vi "Emballae_BDD_Tableau pièces emballées ds GPAO.vi"(8 "error in (no error)":errorcluster caption="entrée d'erreur (pas d'erreur)", 9 "Code bar fixe avec indice":string="1121057400", 11 "connection information":path=path "\\\\Plz-inf-nas\\medic/PARAMETRES_TESTS/PROD_Data-Admin/Connection.udl") -> (0 "error out":errorcluster, 2 "Erreur de\n comunication":bool, 3 "Tableau historique":string[][](array[string])=[["112105740008090004", "01.01.2001 01:01:00", "55", "01234/08-01.01.01", "1", "0"], ["112105740008090006", "01.01.2001 01:01:00", "55", "56789/08-01.01.01", "3", "0"], ["112105740008090007", "01.01.2001 01:01:00", "55", "56789/08-01.01.01", "4", "0"], ["112105740008090007", "01.01.2001 01:01:00", "55", "00123/08-01.01.01", "2", "1"]])   [LabVIEW 2020]
doc: "Renvoie l'historique des articlesidentiques à celui scanné et déjà emballés d'après la GPAO.\nLe tableau historique contient les données suivantes :\n colonne 0 : n° des pièces (code bar 18 chiffres)\n colonne 1 : date\n colonne 2 : visa emballage (n°)\n colonne 3 : n° commande (complet)\n colonne 4 : n° carton\n colonne 5 : n° retour (0, pas un retour)"
uses:
  Modules/FS/60_FS_Controles/60_FS_SetGet.ctl
  <vilib>/addons/database/Connection.llb/DB Tools Open Connec (Path).vi
  <vilib>/addons/database/NI_Database_API.lvlib
panel:
  out "taille(s)":i32
  out "Tableau":string[][](array[string])
  in  "columns com":string[](array[string])=["NO_VALVE", "DATE_EMBALLAGE", "VISA_EMBALLAGE", "NO_COMMANDE", "NO_COMMANDE_LIG", "NO_COMMANDE_LIV", "NO_COMMANDE_VAL", "NO_CARTON", "RETOUR_CLIENT"]
  in  "Table com":string="P_VALIDFLATPROP_M"
  # "0012007703 : F120077"
  # "1121032801 : D3WFIL 417mA 14.4ohm"
  # "5013565504 : F120023 n°Cde tjs égal  0000/0-00.00.00"
  # "0"
  # "1"
  # "2"
  # "3"
  # "4"
  # "5"
  # "6"
  # "7"
  # "8"
  # "9"
  # "0"
  # "1"
  # "2"
  # "3"
  # "4"
  # "5"
  # "6"
  # "7"
  # "8"
  # "9"
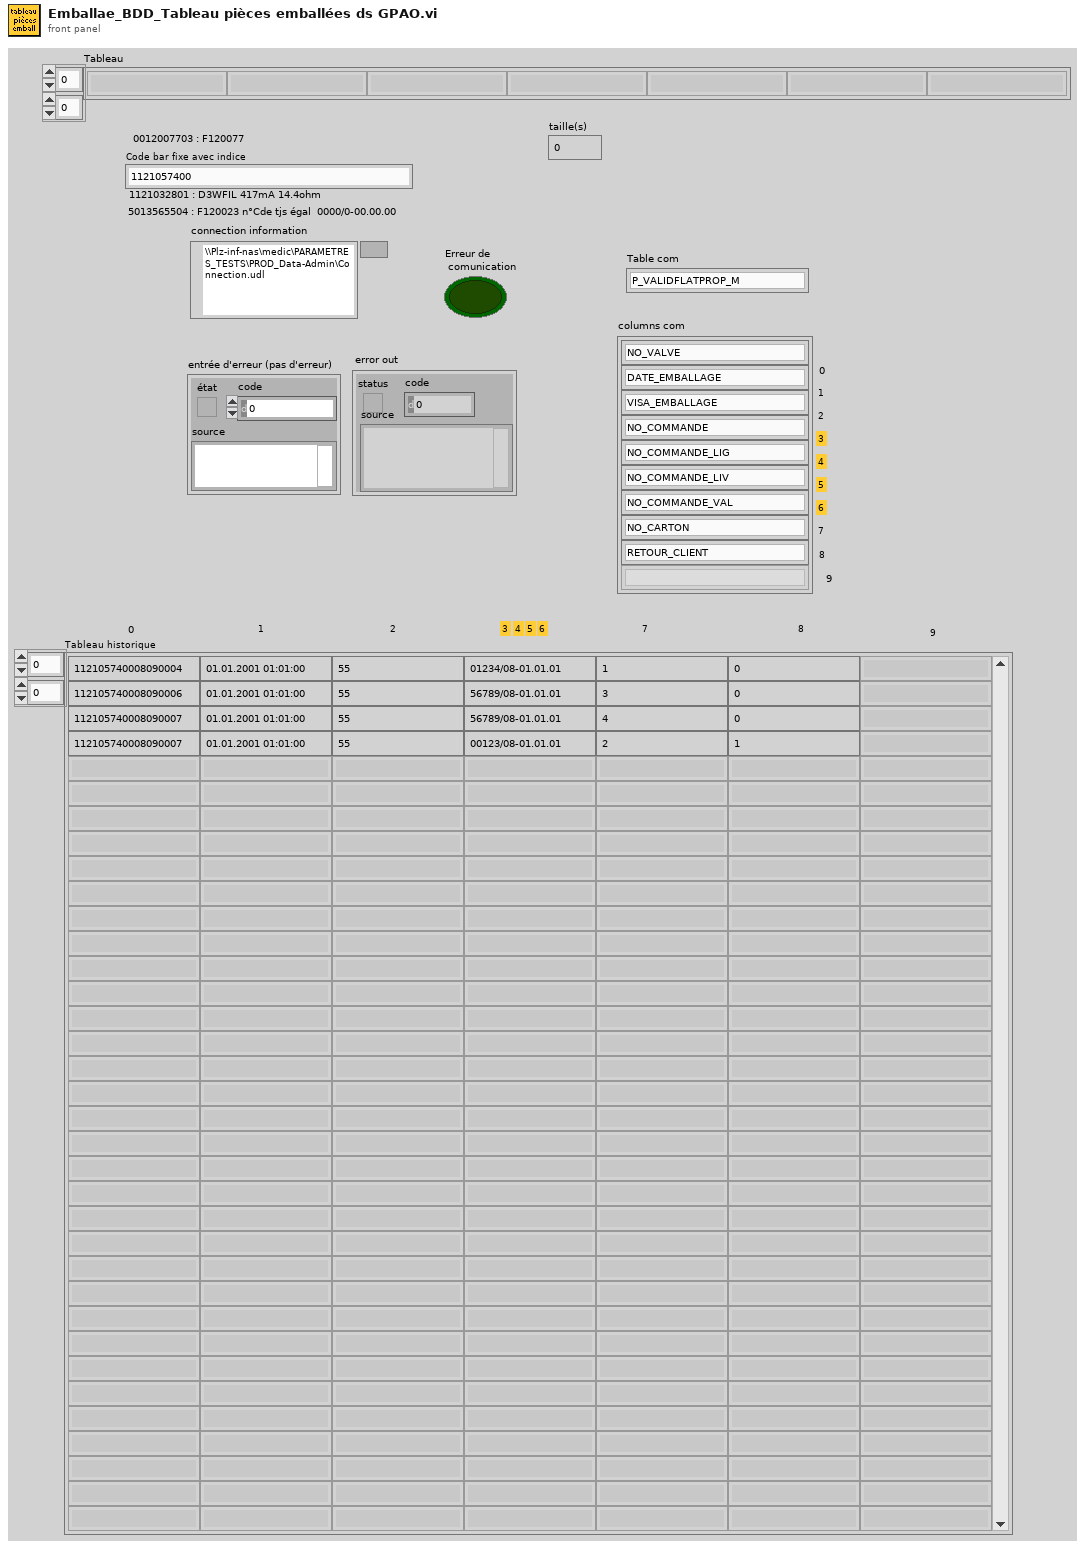
[diagram p1: front panel]
types:
  T1 = typedef "60_FS_SetGet.ctl" = enum16{"set", "get"}
  T2 = typedef "NI_Database_API.lvlib/Conn ObjectReference.ctl" = refnum<k1>
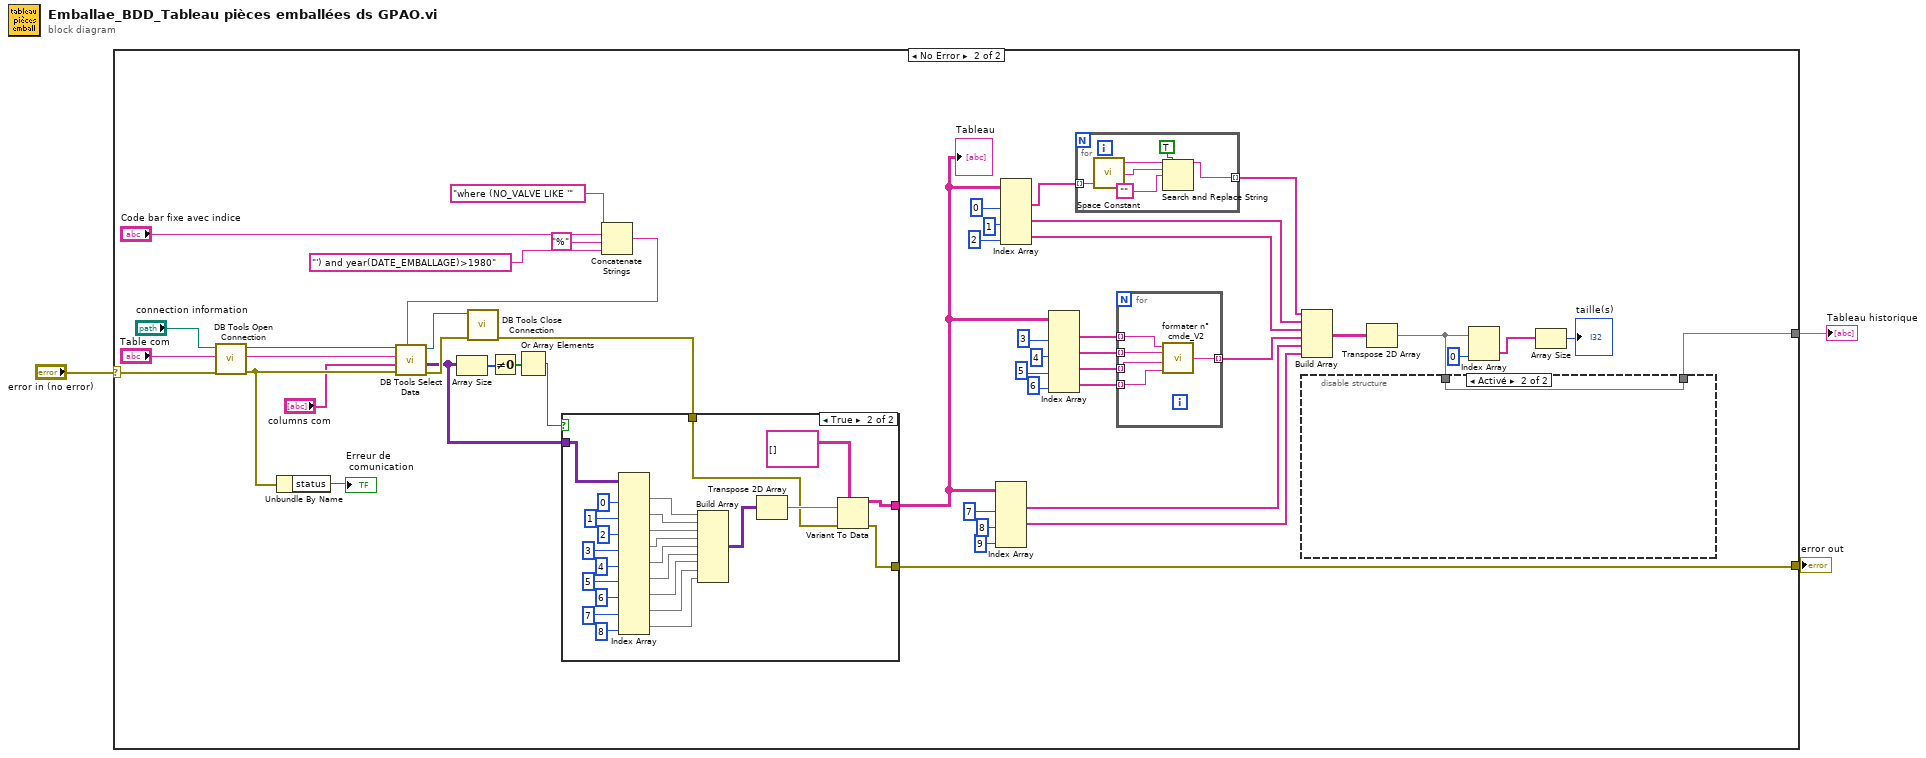
[diagram p0: block diagram]
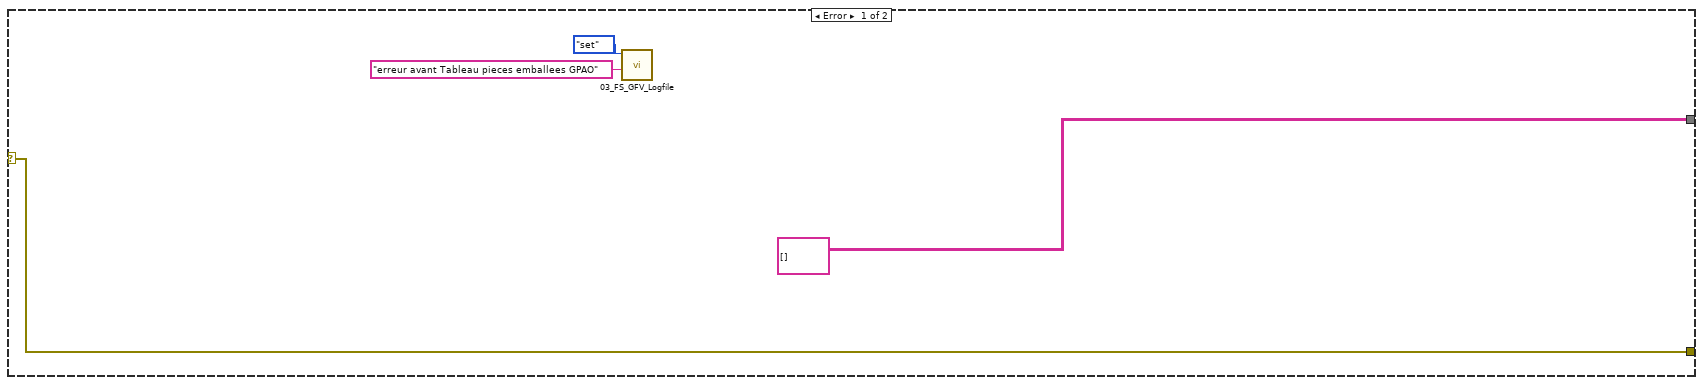
[diagram p2: hidden frame]
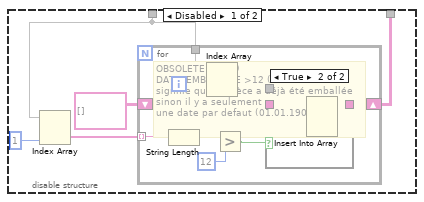
[diagram p3: hidden frame]
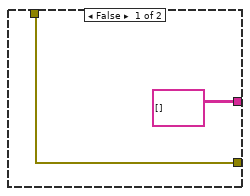
[diagram p5: hidden frame]
diagram:
  n1 = case shown="No Error" "error in (no error)" {
    selector: "error in (no error)" -> [w7 w55]
    tunnel: [w7 w54] -> w3
    tunnel: [string[][] [] w53] -> w2
    frame Error {
      n2 = call "03_FS_GFV_Logfile.vi"("Chaîne"="erreur avant Tableau pieces emballees GPAO", "States"=60_FS_SetGet."set") -> ()  [unwired: 8 in, 2 out]
    }
    frame No Error {
      n3 = call-poly <vilib>:"DB Tools Open Connection.vi"("error in (no error)"=w55, "connection information"="connection information") -> ("error out"=w42:errorcluster, "connection reference"=w51:T2)  [unwired: 6 in]
      n4 = Unbundle By Name(w42) -> ("status"=→"Erreur de\n comunication":bool)
      n5 = Concatenate Strings("where (NO_VALVE LIKE '" ("optional clause"), "Code bar fixe avec indice", "%" ("chaîne"), "') and year(DATE_EMBALLAGE)>1980" ("chaîne")) -> (w38:string)
      n6 = call <vilib>:"DB Tools Select Data.vi"("condition"=w38, "error in (no error)"=w42, "columns"="columns com", "table"="Table com", "connection reference"=w51) -> ("error out"=w46:errorcluster, "data"=w37:variant[][], "connection reference out"=w45:T2)  [unwired: 1 in]
      n7 = Array Size(array=w37) -> (size(s)=w48:i32[])
      n8 = call <vilib>:"DB Tools Close Connection.vi"("error in (no error)"=w46, "connection reference"=w45) -> ("error out"=w43:errorcluster)  [unwired: 5 in]
      n9 = Not Equal To 0?(x=w48) -> (x != 0?=w47:bool[])
      n10 = Or Array Elements(Boolean array=w47) -> (logical OR=w44:bool)
      n11 = case shown="True" w44 {
        tunnel: w37 -> [_ w99]
        tunnel: w43 -> [w86 w101]
        tunnel: [w86 w100] -> w54
        tunnel: [string[][] [] w102] -> w18
        frame False {
        }
        frame True {
          n12 = Index Array(array=w99, index (col) #1=0 ("indice désactivé (col)"), index (col) #2=1 ("indice désactivé (col)"), index (col) #3=2 ("indice désactivé (col)"), index (col) #4=3 ("indice désactivé (col)"), index (col) #5=4 ("indice désactivé (col)"), index (col) #6=5 ("indice désactivé (col)"), index (col) #7=6 ("indice désactivé (col)"), index (col) #8=7 ("indice désactivé (col)"), index (col) #9=8 ("indice désactivé (col)")) -> (element #1=w105:variant[], element #2=w106:variant[], element #3=w111:variant[], element #4=w93:variant[], element #5=w92:variant[], element #6=w91:variant[], element #7=w90:variant[], element #8=w89:variant[], element #9=w87:variant[])  [unwired: 9 in]
          n13 = Build Array(w105, w106, w111, w93, w92, w91, w90, w89, w87) -> (w107:variant[][])
          n14 = Transpose 2D Array(2D array=w107) -> (transposed array=w108:variant[][])
          n15 = Variant To Data(error in=w101, type=string[][] [], Variant=w108) -> (data=w102:string[][], error out=w100:errorcluster)
        }
      }
      "Tableau" <- w18
      n16 = Index Array(array=w18, index (col) #1=7 ("indice désactivé (col)"), index (col) #2=8 ("indice désactivé (col)"), index (col) #3=9 ("indice (col)")) -> (element #1=w17:string[], element #2=w13:string[])  [unwired: 3 in, 1 out]
      n17 = Index Array(array=w18, index (col) #1=0 ("indice désactivé (col)"), index (col) #2=1 ("indice désactivé (col)"), index (col) #3=2 ("indice désactivé (col)")) -> (element #1=w16:string[], element #2=w23:string[], element #3=w22:string[])  [unwired: 3 in]
      n18 = Index Array(array=w18, index (col) #1=3 ("indice désactivé (col)"), index (col) #2=4 ("indice désactivé (col)"), index (col) #3=5 ("indice désactivé (col)"), index (col) #4=6 ("indice désactivé (col)")) -> (element #1=w31:string[], element #2=w30:string[], element #3=w29:string[], element #4=w28:string[])  [unwired: 4 in]
      n19 = for {
        tunnel: w16 -> [w78] mode=indexing
        tunnel: [w75] -> w15 mode=indexing
        n20 = call <vilib>:"Space Constant.vi"() -> ("String"=w77:string)
        n21 = Search and Replace String(replace all?=TRUE ("tout remplacer ? (F)"), input string=w78, search string=w77, replace string="") -> (result string=w75:string)  [unwired: 4 in, 3 out]
      }
      n22 = for {
        tunnel: w31 -> [w84] mode=indexing
        tunnel: w30 -> [w83] mode=indexing
        tunnel: w29 -> [w82] mode=indexing
        tunnel: w28 -> [w81] mode=indexing
        tunnel: [w80] -> w21 mode=indexing
        n23 = call "formater n° cmde_V2.vi"("NO_COMMANDE VAL"=w81, "NO_COMMANDE LIV"=w82, "NO_COMMANDE LIG"=w83, "NO_COMMANDE"=w84) -> ("N° commande"=w80:string)
      }
      n24 = Build Array(w15, w23, w22, w21, w17, w13) -> (w20:string[][])
      n25 = Transpose 2D Array(2D array=w20) -> (transposed array=w12:string[][])
      n26 = disable-structure shown="Activé" {
        disable-tunnel: [w59 w74] -> w53
        disable-tunnel: w12 -> [w56 w74]
        frame Disabled {
          n27 = Index Array(array=w56, index (col)=1 ("indice désactivé (col)")) -> (element=w58:string[])  [unwired: 1 in]
          n28 = for {
            tunnel: w58 -> [w64] mode=indexing
            shift-right: [w69] -> w59
            shift-left: string[][] [] -> [w68]
            tunnel: w56 -> [w67]
            i -> [w66]
            # "OBSOLETE:  (PDA)\nDATE_EMBALLAGE >12 (date + heure)\nsignifie que la pièce a déjà été emballée\nsinon il y a seulement \nune date par defaut (01.01.1904)"
            n29 = String Length(string=w64) -> (length=w63:i32)
            n30 = Index Array(array=w67, index (row)=w66) -> (element=w65:string[])  [unwired: 1 in]
            n31 = Greater?(x=w63, y=12) -> (0:w62:bool)
            n32 = case shown="True" w62 {
              tunnel: [w70 w73] -> w69
              tunnel: w68 -> [w70 w72]
              tunnel: w65 -> [_ w71]
              frame False {
              }
              frame True {
                n33 = Insert Into Array(array=w72, new element=w71) -> (w73:string[][])  [unwired: 2 in]
              }
            }
          }
        }
        frame Enabled {
        }
      }
      n34 = Index Array(array=w12, index (col)=0 ("indice désactivé (col)")) -> (element=w10:string[])  [unwired: 1 in]
      n35 = Array Size(array=w10) -> (size(s)=→"taille(s)":i32)
    }
  }
  "error out" <- w3
  "Tableau historique" <- w2
